vi "DU64_U32SubtractWithBorrow.vi"(2 "y":u32, 3 "x":u32) -> (0 "x - y":u32, 1 "borrow":u32)   [LabVIEW 2020]
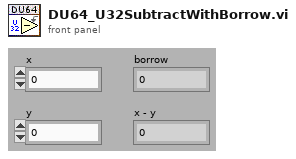
[diagram p1: front panel]
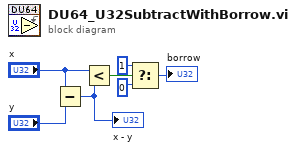
[diagram p0: block diagram]
diagram:
  n1 = Subtract(x="x", y="y") -> (x-y=w6:u32)
  "x - y" <- w6
  n2 = Less?(x="x", y=w6) -> (x < y?=w3:bool)
  n3 = Select(t=u32 1 ("output"), s=w3, f=u32 0 ("output")) -> (s? t:f=→"borrow":u32)
